vi "Get Array Value at Index - 1D Array Double.vi"(8 "error in (no error)":errorcluster, 9 "Default Value if JSON Null":dbl[](array[numeric]), 10 "Index":i32, 11 "JSON Tree In (JSON Array)":variant) -> (0 "error out":errorcluster, 1 "is JSON Null?":bool, 2 "1D Double Array Value":dbl[](array[numeric]), 3 "JSON Tree Out Passthrough":variant)   [LabVIEW 2015, in "i3-json.lvlib"]
doc: "Use this template to build a VI to use as a subVI."
uses:
  i3-json.lvlib
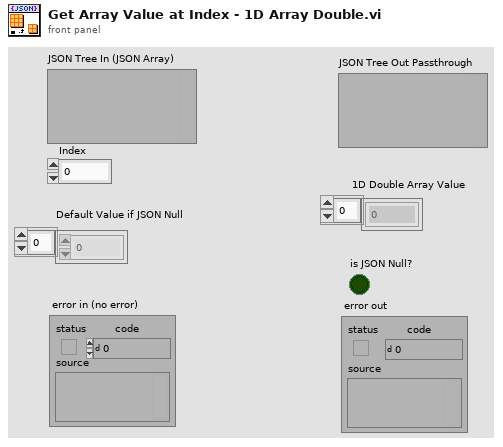
[diagram p1: front panel]
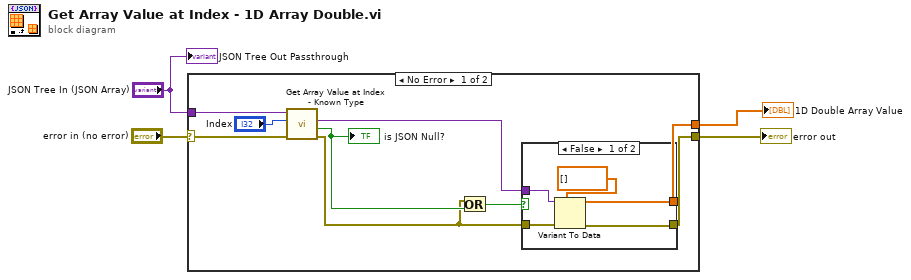
[diagram p0: block diagram]
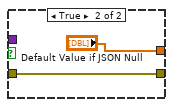
[diagram p2: hidden frame]
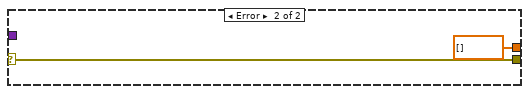
[diagram p3: hidden frame]
diagram:
  n1 = case shown="No Error" "error in (no error)" {
    selector: "error in (no error)" -> [w11 w22]
    tunnel: [w9 w22] -> w3
    tunnel: "JSON Tree In (JSON Array)" -> [w13 _]
    tunnel: [w6 dbl[] [] ("Default Value if JSON Null")] -> w2
    frame No Error {
      n2 = call "Get Array Value at Index - Known Type.vi"("error in (no error)"=w11, "Index"="Index", "JSON Tree In (JSON Array)"=w13) -> ("error out"=w5:errorcluster, "is JSON Null?"=w7:bool, "Value"=w8:variant)  [unwired: 3 in, 3 out]
      "is JSON Null?" <- w7
      n3 = Or(x=w5, y=w7) -> (x .or. y?=w10:bool)
      n4 = case shown="False" w10 {
        tunnel: w5 -> [w18 w20]
        tunnel: [w15 w20] -> w9
        tunnel: w8 -> [w17 _]
        tunnel: [w16 "Default Value if JSON Null"] -> w6
        frame False {
          n5 = Variant To Data(error in=w18, type=dbl[] [], Variant=w17) -> (data=w16:dbl[], error out=w15:errorcluster)
        }
        frame True {
        }
      }
    }
    frame Error {
    }
  }
  "error out" <- w3
  "1D Double Array Value" <- w2
  "JSON Tree Out Passthrough" <- "JSON Tree In (JSON Array)"
